vi "Autonomous No shift 1 Tote 1 Container position 3.vi"() -> ()   [LabVIEW 2014]
uses:
  Autonomous No shift 1 tote 1 container position 3 states.ctl
  Robot Global Data.vi
  Desired Arm Position.vi
  <vilib>/Rock Robotics/WPI/RobotDrive/WPI_RobotDriveGetSetRefNum.vi
  <vilib>/Rock Robotics/WPI/RobotDrive/WPI_RobotDriveArcadeDrive_Standard(NoSaturation).vi
panel:
  out "Enum":T1
  in  "Range":dbl=2.0
  in  "Cluster":T2={"Move Speed"=0.0, "Turning Speed"=0.0, "Arm speed"=0.0, "Desired Arm height (lift)"=15.0, "Initial Turn (Degrees)"=-25.0, "Desired Arm height (lowered)"=0.0, "Drive Forward Time"=0.0, "Turn 90 Degrees"=0.0, "Gyro"=0.0, "Position Speed"=0.3}
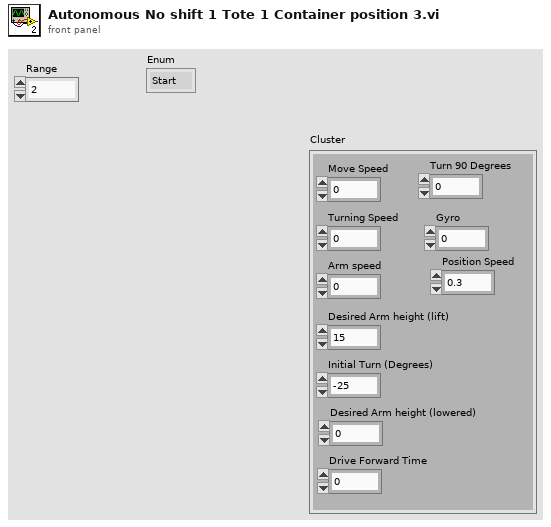
[diagram p1: front panel]
types:
  T1 = typedef "Autonomous No shift 1 tote 1 container position 3 states.ctl" = enum16{"Start", "Grab Container", "Lift Arms", "Move to Position", "Position Robot", "Let go of container + Lower Arms", "Lift tote and container", "Turn 90 degrees", "Move until S.P.", "Stop"}
  T2 = cluster{"Move Speed":dbl, "Turning Speed":dbl, "Arm speed":dbl, "Desired Arm height (lift)":dbl, "Initial Turn (Degrees)":dbl, "Desired Arm height (lowered)":dbl, "Drive Forward Time":dbl, "Turn 90 Degrees":dbl, "Gyro":dbl, "Position Speed":dbl}
  T3 = typedef "WPI_DigitalInputDevRef.ctl" = cluster{"DevStatus":errorcluster, "DIO Channel":T4, "Controller":T5}
  T4 = typedef "FPGA_DIOChannel.ctl" = enum8{"DIO 0", "DIO 1", "DIO 2", "DIO 3", "DIO 4", "DIO 5", "DIO 6", "DIO 7", "DIO 8", "DIO 9", "DIO MXP 0", "DIO MXP 1", "DIO MXP 2", "DIO MXP 3", "DIO MXP 4", "DIO MXP 5", "DIO MXP 6", "DIO MXP 7", "DIO MXP 8", "DIO MXP 9", "DIO MXP 10", "DIO MXP 11", "DIO MXP 12", "DIO MXP 13", "DIO MXP 14", "DIO MXP 15", "Invalid"}
  T5 = typedef "FPGA_TypedefDigitalModule.ctl" = enum16{"Controller 1"}
  T6 = typedef "WPI_RobotDriveDevRef.ctl" = cluster{"DevStatus":errorcluster, "Motors[]":T7[], "Square Inputs":bool, "Max Output":dbl}
  T7 = typedef "WPI_MotorControlDeviceRef.ctl" = cluster{"DeviceStatus":errorcluster, "Type":T8, "PWM":cluster{"Controller":T5, "PWM Channel":T9, "DeadBand":T10}, "CAN":cluster{"Device Number":u8, "Control Mode":T11, "Semaphore":T12, "Max Vout":dbl, "TalonSRX Control Mode":T13}, "Invert":bool, "TransformRef":T14, "InvTransformRef":T14}
  T8 = typedef "WPI_MotorControlType.ctl" = enum16{"PWM", "CAN", "CANTalonSRX"}
  T9 = typedef "FPGA_DIOPWMChannel.ctl" = enum8{"PWM 0", "PWM 1", "PWM 2", "PWM 3", "PWM 4", "PWM 5", "PWM 6", "PWM 7", "PWM 8", "PWM 9", "PWM MXP 0", "PWM MXP 1", "PWM MXP 2", "PWM MXP 3", "PWM MXP 4", "PWM MXP 5", "PWM MXP 6", "PWM MXP 7", "PWM MXP 8", "PWM MXP 9", "Invalid"}
  T10 = typedef "WPI_PWMDeadband.ctl" = cluster{"Name":string, "maxPositivePwm":i32, "minPositivePwm":i32, "centerPwm":i32, "maxNegativePwm":i32, "minNegativePwm":i32, "angularRange":u16}
  T11 = typedef "WPI_CANJaguar_ControlMode.ctl" = enum8{"Percent VBus", "Current", "Speed", "Position", "Voltage"}
  T12 = typedef "Semaphore RefNum" = refnum<k1>
  T13 = typedef "WPI_CANTalonSRX_APIControlMode.ctl" = enum8{"Percent VBus", "Speed", "Position", "Slave", "Unchanged / Invalid"}
  T14 = typedef "WPI_PWMTransform_ConPane.ctl" = refnum<vi>
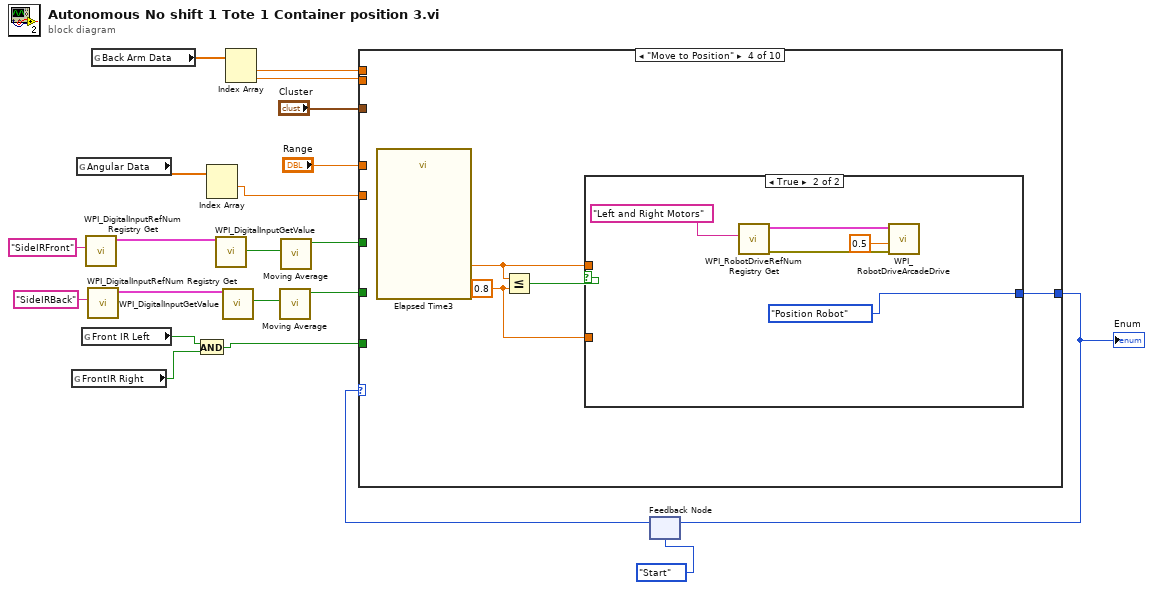
[diagram p0: block diagram]
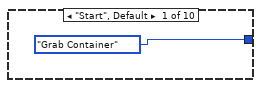
[diagram p2: hidden frame]
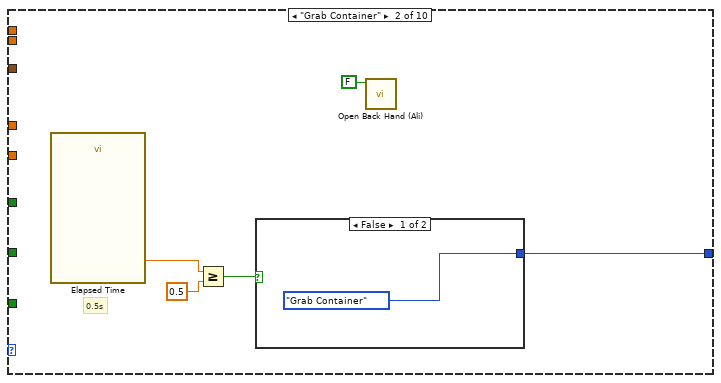
[diagram p3: hidden frame]
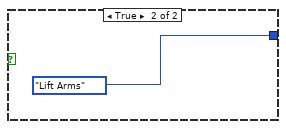
[diagram p4: hidden frame]
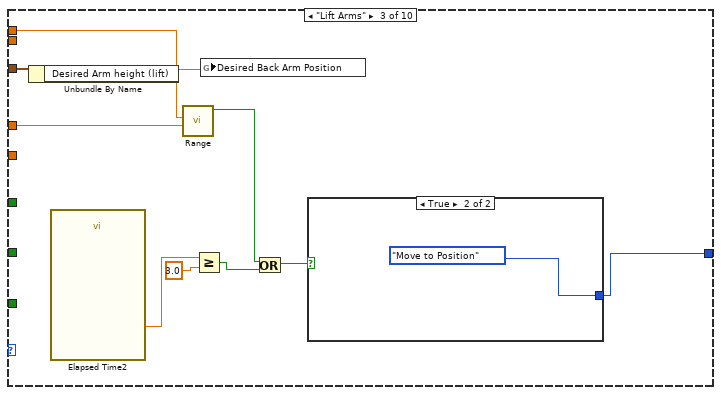
[diagram p5: hidden frame]
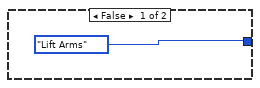
[diagram p6: hidden frame]
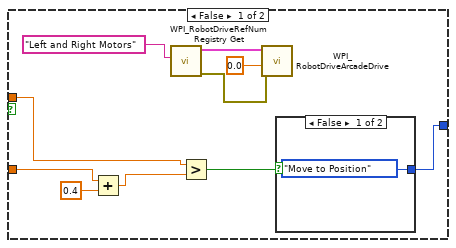
[diagram p7: hidden frame]
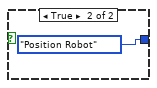
[diagram p8: hidden frame]
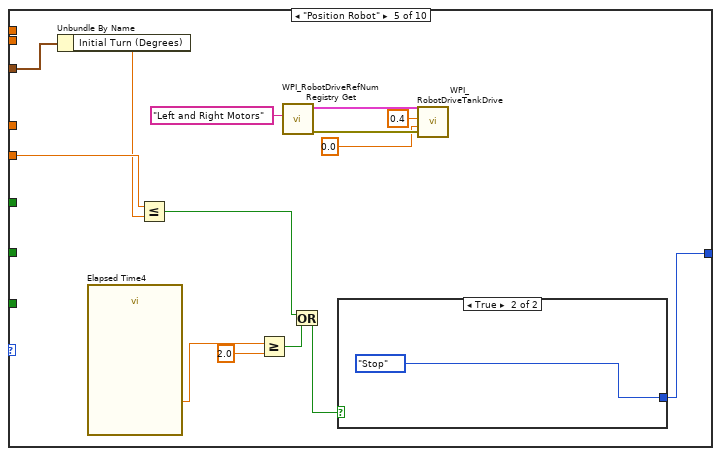
[diagram p9: hidden frame]
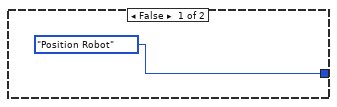
[diagram p10: hidden frame]
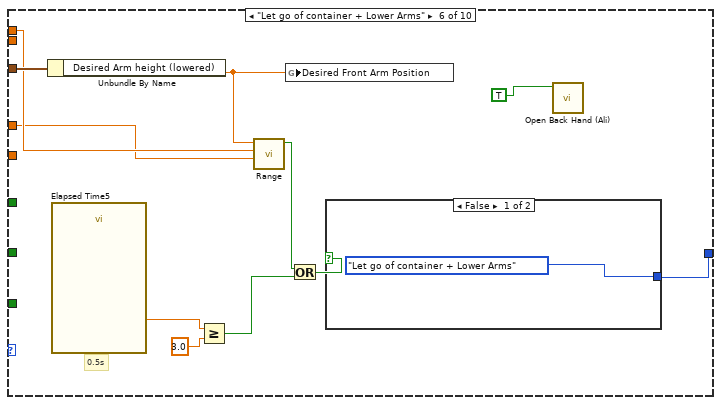
[diagram p11: hidden frame]
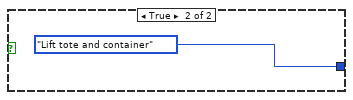
[diagram p12: hidden frame]
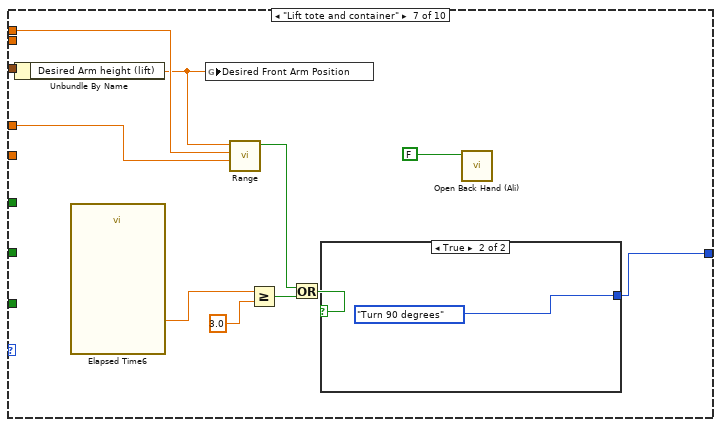
[diagram p13: hidden frame]
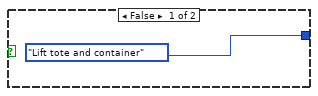
[diagram p14: hidden frame]
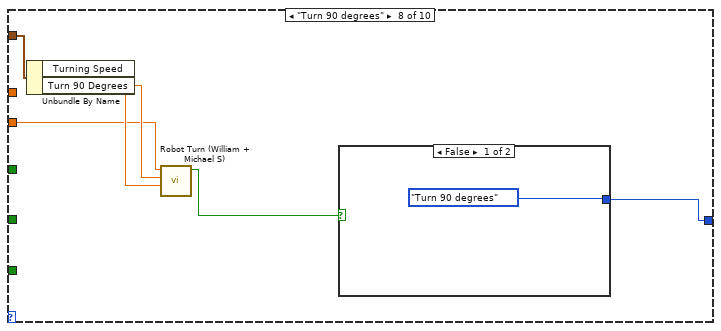
[diagram p15: hidden frame]
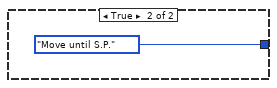
[diagram p16: hidden frame]
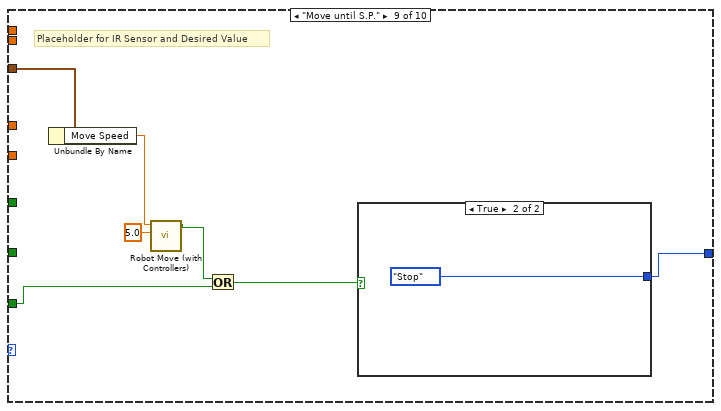
[diagram p17: hidden frame]
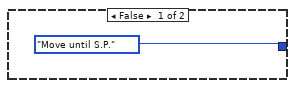
[diagram p18: hidden frame]
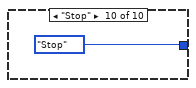
[diagram p19: hidden frame]
diagram:
  n1 = global read "Robot Global Data.vi" "FrontIR Right"() -> (w13:bool)
  n2 = global read "Robot Global Data.vi" "Angular Data"() -> (w17:dbl[])
  n3 = global read "Robot Global Data.vi" "Front IR Left"() -> (w14:bool)
  n4 = call <vilib>:"WPI_DigitalInputRefNum Registry Get.vi"("refnum name"="SideIRFront") -> ("DigitalInputDevRef"=w6:T3)  [unwired: 9 in, 1 out]
  n5 = call <vilib>:"WPI_DigitalInputRefNum Registry Get.vi"("refnum name"="SideIRBack") -> ("DigitalInputDevRef"=w7:T3)  [unwired: 9 in, 1 out]
  n6 = global read "Robot Global Data.vi" "Back Arm Data"() -> (w20:dbl[])
  n7 = And(x=w14, y=w13) -> (x .and. y?=w12:bool)
  n8 = Index Array(array=w17) -> (element #1=w16:dbl)  [unwired: 2 in, 1 out]
  n9 = call <vilib>:"WPI_DigitalInputGetValue.vi"("DigitalInputDevRef"=w6) -> ("Value"=w9:bool)  [unwired: 8 in, 2 out]
  n10 = call <vilib>:"WPI_DigitalInputGetValue.vi"("DigitalInputDevRef"=w7) -> ("Value"=w8:bool)  [unwired: 8 in, 2 out]
  n11 = Index Array(array=w20) -> (element #1=w19:dbl, element #2=w18:dbl)  [unwired: 2 in]
  n12 = call "Moving Average.vi"("Value"=w8) -> ("Moving Boolean Average"=w5:bool)  [unwired: 10 in]
  n13 = call "Moving Average.vi"("Value"=w9) -> ("Moving Boolean Average"=w4:bool)  [unwired: 10 in]
  n14 = feedback #1(Autonomous_No_shift_1_tote_1_container_position_3_states."Start") -> (w3:T1)
  n15 = case shown="\"Move to Position\"" w3 {
    tunnel: "Cluster" -> [_ _ w32 _ w74 w83 w96 w110 w115 _]
    tunnel: [Autonomous_No_shift_1_tote_1_container_position_3_states."Grab Container" w23 w30 w42 w73 w84 w97 w106 w118 Autonomous_No_shift_1_tote_1_container_position_3_states."Stop"] -> w1
    tunnel: w12 -> [_ _ _ _ _ _ _ _ w117 _]
    tunnel: w19 -> [_ _ w35 _ _ w82 w95 _ _ _]
    tunnel: w18 -> [_ _ _ _ _ _ _ _ _ _]
    tunnel: w16 -> [_ _ _ _ w69 _ _ w105 _ _]
    tunnel: "Range" -> [_ _ w33 _ _ w79 w92 _ _ _]
    tunnel: w5 -> [_ _ _ _ _ _ _ _ _ _]
    tunnel: w4 -> [_ _ _ _ _ _ _ _ _ _]
    frame "Start", Default {
    }
    frame "Grab Container" {
      # "0.5s"
      n16 = call "Elapsed Time"() -> ("Elapsed Time (s)"=w27:dbl)  [unwired: 12 in, 7 out]
      n17 = Greater Or Equal?(x=w27, y=0.5) -> (x >= y?=w25:bool)
      n18 = case shown="False" w25 {
        tunnel: [Autonomous_No_shift_1_tote_1_container_position_3_states."Grab Container" Autonomous_No_shift_1_tote_1_container_position_3_states."Lift Arms"] -> w23
        frame False {
        }
        frame True {
        }
      }
      n19 = call "Open Back Hand (Ali).vi"("Open?"=FALSE) -> ()  [unwired: 11 in]
    }
    frame "Lift Arms" {
      n20 = Unbundle By Name(w32) -> ("Desired Arm height (lift)"=w31:dbl)
      n21 = call "Elapsed Time2"() -> ("Elapsed Time (s)"=w39:dbl)  [unwired: 12 in, 7 out]
      n22 = call "Range.vi"("Range"=w33, "Input"=w35) -> ("In Range?"=w34:bool)  [unwired: 9 in]
      n23 = Greater Or Equal?(x=w39, y=3.0) -> (x >= y?=w37:bool)
      n24 = global write "Desired Arm Position.vi" "Desired Back Arm Position"(w31) -> ()
      n25 = Or(x=w34, y=w37) -> (x .or. y?=w36:bool)
      n26 = case shown="True" w36 {
        tunnel: [Autonomous_No_shift_1_tote_1_container_position_3_states."Lift Arms" Autonomous_No_shift_1_tote_1_container_position_3_states."Move to Position"] -> w30
        frame False {
        }
        frame True {
        }
      }
    }
    frame "Move to Position" {
      w43 = 0.8 ("y")
      n27 = call "Elapsed Time3"() -> ("Elapsed Time (s)"=w44:dbl)  [unwired: 12 in, 7 out]
      n28 = Less Or Equal?(x=w44, y=w43) -> (x <= y?=w45:bool)
      n29 = case shown="True" w45 {
        tunnel: w44 -> [w51 _]
        tunnel: w43 -> [w49 _]
        tunnel: [w46 Autonomous_No_shift_1_tote_1_container_position_3_states."Position Robot"] -> w42
        frame False {
          n30 = Add(x=w49, y=0.4) -> (x+y=w47:dbl)
          n31 = call <vilib>:"WPI_RobotDriveRefNum Registry Get.vi"("refnum name"="Left and Right Motors") -> ("error out"=w54:errorcluster, "RobotDriveDevRef"=w52:T6)  [unwired: 9 in]
          n32 = Greater?(x=w51, y=w47) -> (0:w50:bool)
          n33 = call-poly <vilib>:"WPI_RobotDriveArcadeDrive.vi"("error in (no error)"=w54, "Y axis value"=0.0, "RobotDriveDevRef"=w52) -> ()  [unwired: 6 in, 3 out]
          n34 = case shown="False" w50 {
            tunnel: [Autonomous_No_shift_1_tote_1_container_position_3_states."Move to Position" Autonomous_No_shift_1_tote_1_container_position_3_states."Position Robot"] -> w46
            frame False {
            }
            frame True {
            }
          }
        }
        frame True {
          n35 = call <vilib>:"WPI_RobotDriveRefNum Registry Get.vi"("refnum name"="Left and Right Motors") -> ("error out"=w61:errorcluster, "RobotDriveDevRef"=w62:T6)  [unwired: 9 in]
          n36 = call-poly <vilib>:"WPI_RobotDriveArcadeDrive.vi"("error in (no error)"=w61, "Y axis value"=0.5, "RobotDriveDevRef"=w62) -> ()  [unwired: 6 in, 3 out]
        }
      }
    }
    frame "Position Robot" {
      n37 = Unbundle By Name(w74) -> ("Initial Turn (Degrees)"=w68:dbl)
      n38 = call "Elapsed Time4"() -> ("Elapsed Time (s)"=w76:dbl)  [unwired: 12 in, 7 out]
      n39 = Less Or Equal?(x=w69, y=w68) -> (x <= y?=w66:bool)
      n40 = Greater Or Equal?(x=w76, y=2.0) -> (x >= y?=w67:bool)
      n41 = call <vilib>:"WPI_RobotDriveRefNum Registry Get.vi"("refnum name"="Left and Right Motors") -> ("error out"=w71:errorcluster, "RobotDriveDevRef"=w72:T6)  [unwired: 9 in]
      n42 = Or(x=w66, y=w67) -> (x .or. y?=w65:bool)
      n43 = case shown="True" w65 {
        tunnel: [Autonomous_No_shift_1_tote_1_container_position_3_states."Position Robot" Autonomous_No_shift_1_tote_1_container_position_3_states."Stop"] -> w73
        frame False {
        }
        frame True {
        }
      }
      n44 = call <vilib>:"WPI_RobotDriveTankDrive.vi"("error in (no error)"=w71, "Right axis value"=0.0 ("Left axis value"), "Left axis value"=0.4, "RobotDriveDevRef"=w72) -> ()  [unwired: 5 in, 3 out]
    }
    frame "Let go of container + Lower Arms" {
      # "0.5s"
      n45 = Unbundle By Name(w83) -> ("Desired Arm height (lowered)"=w81:dbl)
      n46 = call "Elapsed Time5"() -> ("Elapsed Time (s)"=w87:dbl)  [unwired: 12 in, 7 out]
      n47 = Greater Or Equal?(x=w87, y=3.0) -> (x >= y?=w89:bool)
      n48 = call "Range.vi"("Range"=w79, "Input"=w82, "In Range of"=w81) -> ("In Range?"=w80:bool)  [unwired: 8 in]
      n49 = global write "Desired Arm Position.vi" "Desired Front Arm Position"(w81) -> ()
      n50 = Or(x=w80, y=w89) -> (x .or. y?=w85:bool)
      n51 = case shown="False" w85 {
        tunnel: [Autonomous_No_shift_1_tote_1_container_position_3_states."Let go of container + Lower Arms" Autonomous_No_shift_1_tote_1_container_position_3_states."Lift tote and container"] -> w84
        frame False {
        }
        frame True {
        }
      }
      n52 = call "Open Back Hand (Ali).vi"("Open?"=TRUE) -> ()  [unwired: 11 in]
    }
    frame "Lift tote and container" {
      n53 = Unbundle By Name(w96) -> ("Desired Arm height (lift)"=w94:dbl)
      n54 = call "Elapsed Time6"() -> ("Elapsed Time (s)"=w101:dbl)  [unwired: 12 in, 7 out]
      n55 = global write "Desired Arm Position.vi" "Desired Front Arm Position"(w94) -> ()
      n56 = call "Range.vi"("Range"=w92, "Input"=w95, "In Range of"=w94) -> ("In Range?"=w93:bool)  [unwired: 8 in]
      n57 = Greater Or Equal?(x=w101, y=3.0) -> (x >= y?=w99:bool)
      n58 = Or(x=w93, y=w99) -> (x .or. y?=w98:bool)
      n59 = case shown="True" w98 {
        tunnel: [Autonomous_No_shift_1_tote_1_container_position_3_states."Lift tote and container" Autonomous_No_shift_1_tote_1_container_position_3_states."Turn 90 degrees"] -> w97
        frame False {
        }
        frame True {
        }
      }
      n60 = call "Open Back Hand (Ali).vi"("Open?"=FALSE) -> ()  [unwired: 11 in]
    }
    frame "Turn 90 degrees" {
      n61 = Unbundle By Name(w110) -> ("Turning Speed"=w109:dbl, "Turn 90 Degrees"=w108:dbl)
      n62 = call "Robot Turn (William + Michael S).vi"("X axis value"=w109, "Desired Degree"=w108, "Gyro Degrees"=w105) -> ("Stop"=w107:bool)  [unwired: 8 in]
      n63 = case shown="False" w107 {
        tunnel: [Autonomous_No_shift_1_tote_1_container_position_3_states."Turn 90 degrees" Autonomous_No_shift_1_tote_1_container_position_3_states."Move until S.P."] -> w106
        frame False {
        }
        frame True {
        }
      }
    }
    frame "Move until S.P." {
      # "Placeholder for IR Sensor and Desired Value"
      n64 = Unbundle By Name(w115) -> ("Move Speed"=w114:dbl)
      n65 = call "Robot Move (with Controllers).vi"("Time Target (s)"=5.0, "Speed"=w114) -> ("Stop"=w116:bool)  [unwired: 9 in]
      n66 = Or(x=w116, y=w117) -> (x .or. y?=w119:bool)
      n67 = case shown="True" w119 {
        tunnel: [Autonomous_No_shift_1_tote_1_container_position_3_states."Move until S.P." Autonomous_No_shift_1_tote_1_container_position_3_states."Stop"] -> w118
        frame False {
        }
        frame True {
        }
      }
    }
    frame "Stop" {
    }
  }
  "Enum" <- w1
  n68 = feedback-in #1(w1) -> ()
